vi "align single V1.0.vi"(8 "error in (no error)":errorcluster, 10 "Target (Volt)":dbl) -> (0 "error out":errorcluster)   [LabVIEW 2019]
uses:
  <vilib>/Platform/TimedLoop/XDataNode/timing_clust.ctl
  <vilib>/Platform/TimedLoop/XDataNode/nitl_modes.ctl
  <vilib>/Platform/TimedLoop/XDataNode/wakeup.ctl
  <vilib>/addons/control/pid/pid.llb/PID (DBL).vi
  <vilib>/platform/TimedLoop/XDataNode/XDataNode.xnode
  <vilib>/Platform/TimedLoop/XDataNode/XDNodeRunTimeDep.lvlib
  <vilib>/addons/control/pid/NI_PID_pid.lvlib
panel:
  out "Waveform Chart 2":dbl(graph)
  out "Waveform Chart":dbl(graph)
  in  "stop":bool
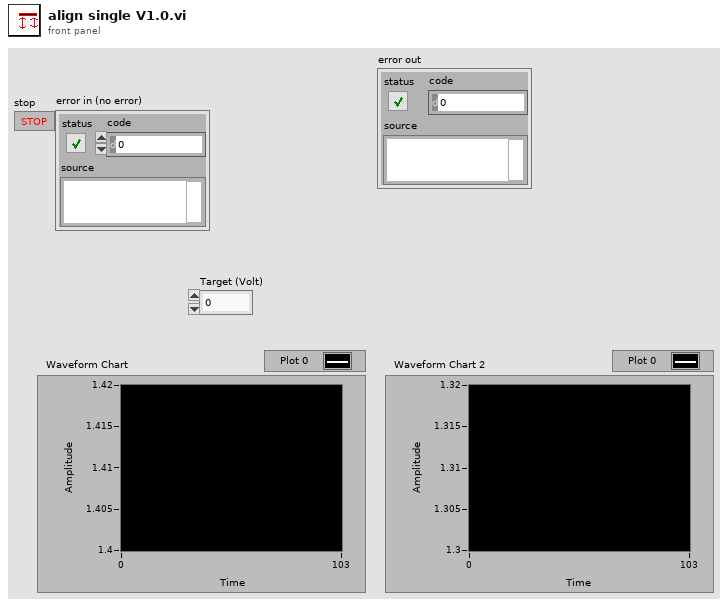
[diagram p1: front panel]
types:
  T1 = typedef "XDNodeRunTimeDep.lvlib/timing_clust.ctl" = cluster{"Expected End [f-1]":u64, "Actual End [f-1]":u64, "Finished Late? [f-1]":bool, "Expected End [i-1]":u64, "Actual End [i-1]":u64, "Finished Late? [i-1]":bool, "Expected Start [i]":u64, "Actual Start [i]":u64, "Expected Start [f]":u64, "Actual Start [f]":u64, "Source Name":string, "Structure Name":string, "Period":i64, "Deadline":i64, "Offset":i64, "Start":i64, "Priority":i32, "Timeout":i32, "Mode":T2, "Wakeup Reason":T3, "Error":errorcluster, "Source Type":string, "Secondary Source Type":string, "Global End Time":u64, "Global Start Time":u64, "Frame Duration":u64, "Iteration Duration":u64, "Assigned CPU":i32, "I/O Scan Engine Mode":u32}
  T2 = typedef "XDNodeRunTimeDep.lvlib/nitl_modes.ctl" = enum32{"No Change", "Process missed periods, maintain original phase", "Discard missed periods, maintain original phase", "Process missed periods, ignore original phase", "Discard missed periods, ignore original phase"}
  T3 = typedef "XDNodeRunTimeDep.lvlib/wakeup.ctl" = enum32{"Normal", "Aborted", "Asynchronous wakeup", "Timing source error", "Timed loop error", "Timeout"}
  T4 = typedef "IR out.ctl" = cluster{"DC estimate (V) 2":dbl, "DC estimate (V)":dbl, "AC estimate (Vrms)":dbl, "AC estimate (Vrms) 2":dbl}
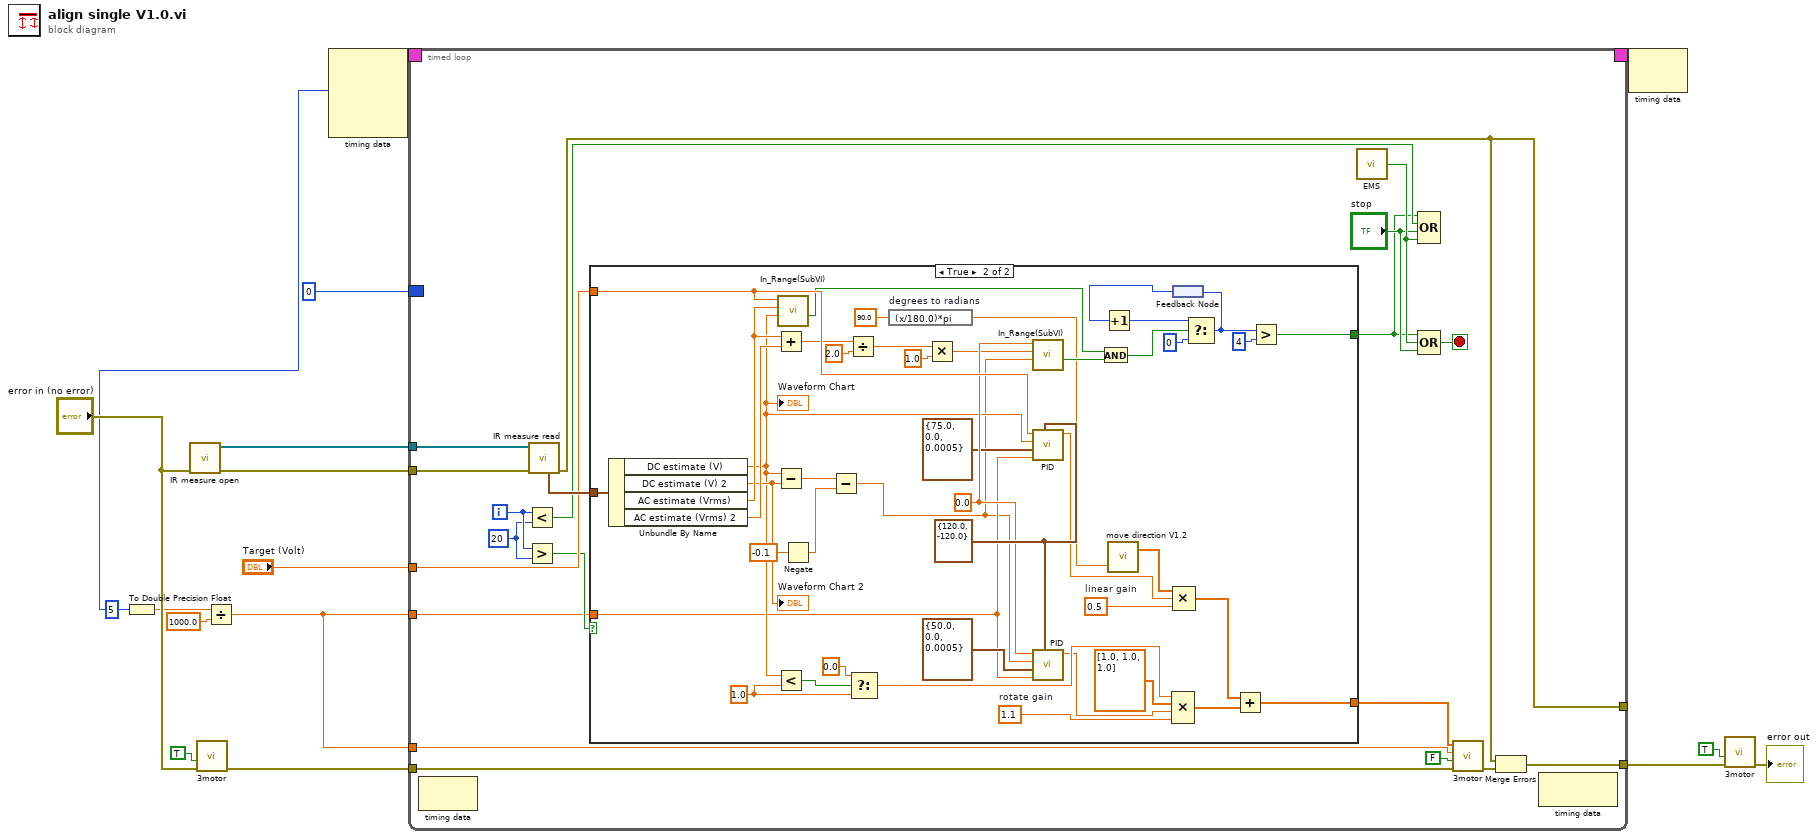
[diagram p0: block diagram]
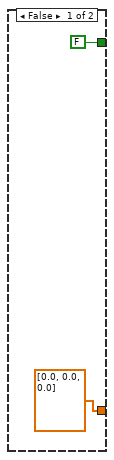
[diagram p2: hidden frame]
diagram:
  w5 = i64 5 ("Period")
  n1 = To Double Precision Float(number=w5) -> (double precision float=w4:dbl)
  n2 = call "IR measure open.vi"("error in (no error)"="error in (no error)") -> ("error out"=w13:errorcluster, "ref array"=w14:refnum<class "IR sensor.lvclass">[])  [unwired: 9 in]
  n3 = call "3motor.vi"("error in (no error)"="error in (no error)", "Reset"=TRUE) -> ("error out"=w10:errorcluster)  [unwired: 8 in, 1 out]
  n4 = Divide(x=w4, y=1000.0) -> (x/y=w1:dbl)
  n5 = node-c288(w5) -> (w16:T1)  [unwired: 3 in]
  n6 = timed-loop {
    timing: w16 -> [_]
    timing-out: [_] -> w15
    tunnel: w14 -> [w36]
    tunnel: [w17] -> _
    tunnel: w13 -> [w35]
    tunnel: "Target (Volt)" -> [w33]
    tunnel: [w18] -> w11
    tunnel: w10 -> [w31]
    tunnel: w1 -> [w29]
    border: 0 -> [_]
    tunnel: w1 -> [w23]
    i -> [w27]
    stop <- w22 stop-if-true
    w26 = 20 ("y")
    n7 = node-c288() -> ()  [unwired: 1 in, 1 out]
    n8 = Less?(x=w27, y=w26) -> (x < y?=w30:bool)
    n9 = Greater?(x=w27, y=w26) -> (0:w25:bool)
    n10 = call "IR measure read.vi"("error in (no error)"=w35, "ref array"=w36) -> ("error out"=w17:errorcluster, "output cluster"=w34:T4)  [unwired: 7 in, 1 out]
    n11 = case shown="True" w25 {
      tunnel: w34 -> [_ w82]
      tunnel: w33 -> [_ w81]
      tunnel: [FALSE w60] -> w19
      tunnel: [dbl[] [0.0, 0.0, 0.0] w66] -> w28
      tunnel: w23 -> [_ w45]
      frame False {
      }
      frame True {
        w54 = 1.0 ("y")
        w80 = 0.5  # linear gain
        w69 = 1.1  # rotate gain
        w77 = 0.0 ("Setpoint")
        w79 = cluster{"output high":dbl, "output low":dbl} {"output high"=120.0, "output low"=-120.0} ("output range")
        n12 = Unbundle By Name(w82) -> ("DC estimate (V)"=w48:dbl, "DC estimate (V) 2"=w61:dbl, "AC estimate (Vrms)"=w76:dbl, "AC estimate (Vrms) 2"=w75:dbl)
        "Waveform Chart" <- w48
        "Waveform Chart 2" <- w61
        n13 = Add(x=w76, y=w75) -> (x+y=w74:dbl)
        n14 = Subtract(x=w48, y=w61) -> (x-y=w43:dbl)
        n15 = Less?(x=w48, y=w54) -> (x < y?=w56:bool)
        n16 = call "In_Range(SubVI).vi"("Proccess Variable"=w48, "AC estimate (Vrms)"=w76, "Setpoint"=w81) -> ("In Range?"=w59:bool)  [unwired: 7 in, 1 out]
        n17 = Negate(x=-0.1 ("align offset")) -> (-x=w42:dbl)
        n18 = Subtract(x=w43, y=w42) -> (x-y=w44:dbl)
        n19 = Divide(x=w74, y=2.0) -> (x/y=w72:dbl)
        n20 = Select(t=0.0, s=w56, f=w54) -> (s? t:f=w53:dbl)
        n21 = expression code="(x/180.0)*pi" "degrees to radians"(90.0) -> (w40:dbl)
        n22 = Multiply(x=w72, y=1.0) -> (x*y=w52:dbl)
        n23 = call "In_Range(SubVI).vi"("Proccess Variable"=w44, "AC estimate (Vrms)"=w52, "Setpoint"=w77) -> ("In Range?"=w58:bool)  [unwired: 7 in, 1 out]
        n24 = call-poly <vilib>:"PID.vi"("output range"=w79, "dt (s)"=w45, "PID gains"=cluster{"Kp":dbl, "Ki":dbl, "Kd":dbl} {"Kp"=75.0, "Ki"=0.0, "Kd"=0.0005} ("PID"), "process variable"=w48, "setpoint"=w81) -> ("output"=w47:dbl)  [unwired: 5 in, 1 out]
        n25 = call-poly <vilib>:"PID.vi"("output range"=w79, "dt (s)"=w45, "PID gains"=cluster{"Kp":dbl, "Ki":dbl, "Kd":dbl} {"Kp"=50.0, "Ki"=0.0, "Kd"=0.0005} ("PID"), "process variable"=w44, "setpoint"=w77) -> ("output"=w46:dbl)  [unwired: 5 in, 1 out]
        n26 = And(x=w59, y=w58) -> (x .and. y?=w57:bool)
        n27 = call "move direction V1.2.vi"("theta"=w40) -> ("out array"=w39:dbl[])  [unwired: 1 in, 1 out]
        n28 = Compound Arithmetic op=MULTIPLY(w53, dbl[] [1.0, 1.0, 1.0], w46, w69) -> (w67:dbl[])
        n29 = feedback #1() -> (w64:i32)
        n30 = Increment(x=w64) -> (x+1=w65:i32)
        n31 = Compound Arithmetic op=MULTIPLY(w39, w47, w80) -> (w68:dbl[])
        n32 = Select(t=w65, s=w57, f=0) -> (s? t:f=w63:i32)
        n33 = feedback-in #1(w63) -> ()
        n34 = Add(x=w68, y=w67) -> (x+y=w66:dbl[])
        n35 = Greater?(x=w63, y=4) -> (0:w60:bool)
      }
    }
    n36 = call "EMS.vi"() -> ("A/DIO4 (Pin 19)"=w24:bool)
    n37 = Compound Arithmetic op=OR(w19, w30, "stop", w24) -> ()  [unwired: 1 out]
    n38 = Compound Arithmetic op=OR(w19, w24, "stop") -> (w22:bool)
    n39 = call "3motor.vi"("error in (no error)"=w31, "Reset"=FALSE, "dt(s)"=w29, "Motor speed"=w28) -> ("error out"=w32:errorcluster)  [unwired: 6 in, 1 out]
    n40 = Merge Errors(w17, w32) -> (w18:errorcluster)
    n41 = node-c288() -> ()  [unwired: 1 in, 1 out]
  }
  n42 = node-c288(w15) -> ()  [unwired: 1 out]
  n43 = call "3motor.vi"("error in (no error)"=w11, "Reset"=TRUE) -> ("error out"=→"error out":errorcluster)  [unwired: 8 in, 1 out]
